vi "TriEdges-Box intersection test.vi"(1 "Triangle":T1, 2 "Box":T2={"Face 0"={"V0"=[], "V1"=[], "V2"=[], "V3"=[], "E0"=[], "E1"=[], "E2"=[], "E3"=[], "n^"=[], "nE0^"=[], "nE1^"=[], "nE2^"=[], "nE3^"=[]}, "Face 1"={"V0"=[], "V1"=[], "V2"=[], "V3"=[], "E0"=[], "E1"=[], "E2"=[], "E3"=[], "n^"=[], "nE0^"=[], "nE1^"=[], "nE2^"=[], "nE3^"=[]}, "Face 2"={"V0"=[], "V1"=[], "V2"=[], "V3"=[], "E0"=[], "E1"=[], "E2"=[], "E3"=[], "n^"=[], "nE0^"=[], "nE1^"=[], "nE2^"=[], "nE3^"=[]}, "Face 3"={"V0"=[], "V1"=[], "V2"=[], "V3"=[], "E0"=[], "E1"=[], "E2"=[], "E3"=[], "n^"=[], "nE0^"=[], "nE1^"=[], "nE2^"=[], "nE3^"=[]}, "Face 4"={"V0"=[], "V1"=[], "V2"=[], "V3"=[], "E0"=[], "E1"=[], "E2"=[], "E3"=[], "n^"=[], "nE0^"=[], "nE1^"=[], "nE2^"=[], "nE3^"=[]}, "Face 5"={"V0"=[], "V1"=[], "V2"=[], "V3"=[], "E0"=[], "E1"=[], "E2"=[], "E3"=[], "n^"=[], "nE0^"=[], "nE1^"=[], "nE2^"=[], "nE3^"=[]}, "Level"=-1, "Pmax"=[], "Pmin"=[], "Parent"=-1, "Child 1"=-1, "Child 2"=-1, "Child 3"=-1, "Child 4"=-1, "Child 5"=-1, "Child 6"=-1, "Child 7"=-1, "Child 8"=-1, "Triangles"=[], "is leaf node"=FALSE}) -> (0 "Intersection":bool)   [LabVIEW 2014]
uses:
  Typedefs/TreeNodeBox.ctl
  Typedefs/Quad.ctl
  Typedefs/Triangle.ctl
panel:
  # "PN 17/01/2015"
  # "Vertices"
  # "Edges"
  # "Unit normal"
  # "pre-store"
  # "Vertices"
  # "Edges"
  # "Unit normal"
  # "Edge unit normals"
  # "Vertices"
  # "Edges"
  # "Unit normal"
  # "Edge unit normals"
  # "Vertices"
  # "Edges"
  # "Unit normal"
  # "Edge unit normals"
  # "Vertices"
  # "Edges"
  # "Unit normal"
  # "Edge unit normals"
  # "Vertices"
  # "Edges"
  # "Unit normal"
  # "Edge unit normals"
  # "Vertices"
  # "Edges"
  # "Unit normal"
  # "Edge unit normals"
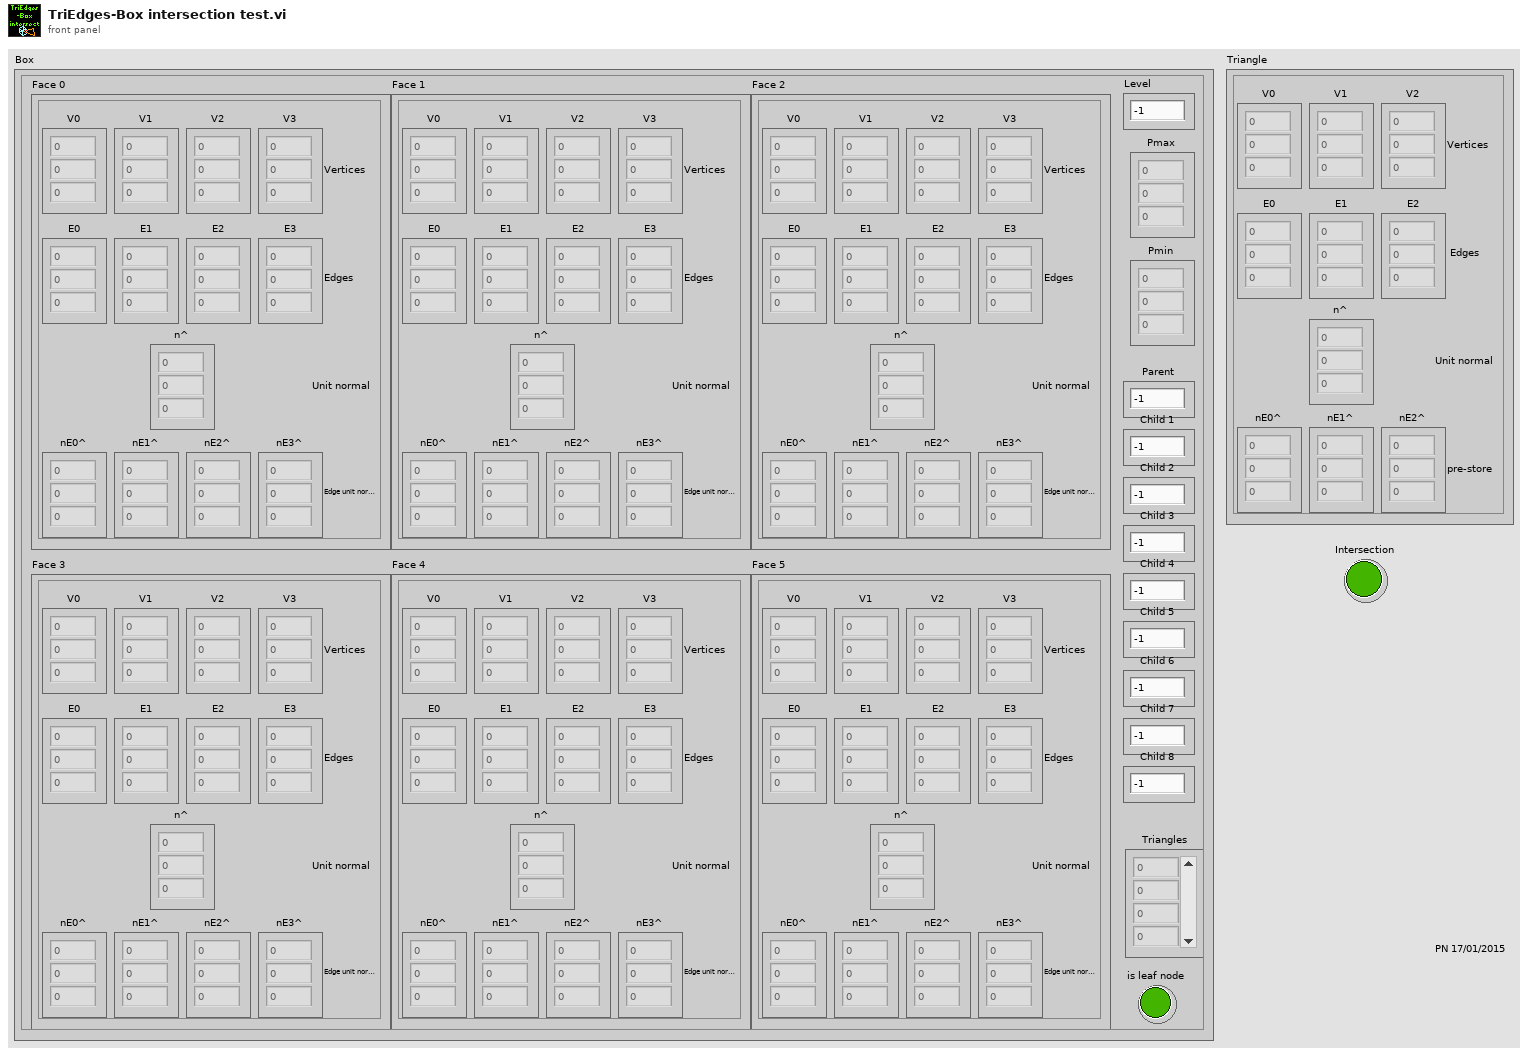
[diagram p1: front panel]
types:
  T1 = typedef "Triangle.ctl" = cluster{"V0":sgl[], "V1":sgl[], "V2":sgl[], "E0":sgl[], "E1":sgl[], "E2":sgl[], "n^":sgl[], "nE0^":sgl[], "nE1^":sgl[], "nE2^":sgl[]}
  T2 = typedef "TreeNodeBox.ctl" = cluster{"Face 0":T3, "Face 1":T3, "Face 2":T3, "Face 3":T3, "Face 4":T3, "Face 5":T3, "Level":i32, "Pmax":sgl[], "Pmin":sgl[], "Parent":i32, "Child 1":i32, "Child 2":i32, "Child 3":i32, "Child 4":i32, "Child 5":i32, "Child 6":i32, "Child 7":i32, "Child 8":i32, "Triangles":i32[], "is leaf node":bool}
  T3 = typedef "Quad.ctl" = cluster{"V0":sgl[], "V1":sgl[], "V2":sgl[], "V3":sgl[], "E0":sgl[], "E1":sgl[], "E2":sgl[], "E3":sgl[], "n^":sgl[], "nE0^":sgl[], "nE1^":sgl[], "nE2^":sgl[], "nE3^":sgl[]}
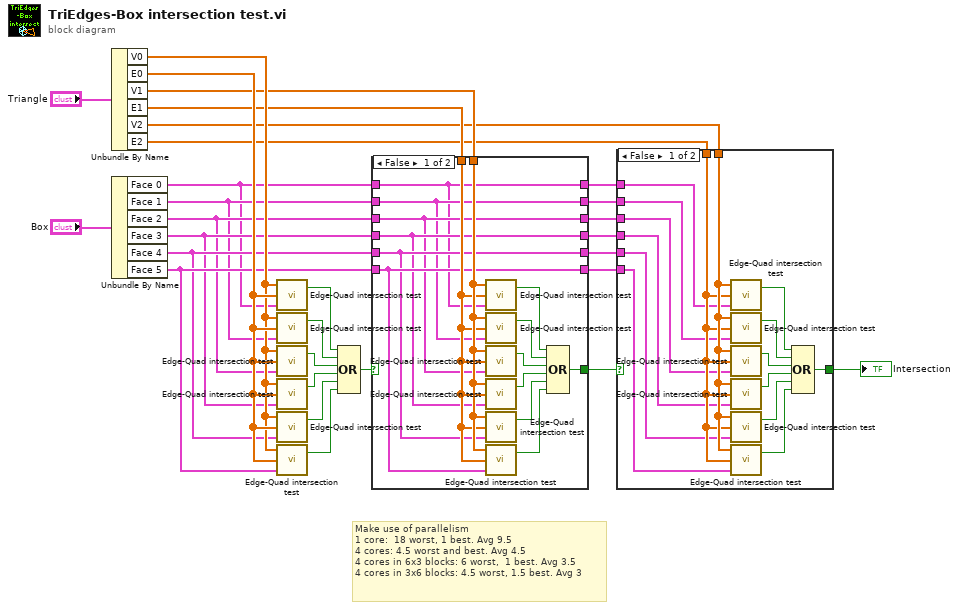
[diagram p0: block diagram]
diagram:
  # "Make use of parallelism\n1 core:  18 worst, 1 best. Avg 9.5\n4 cores: 4.5 worst and best. Avg 4.5\n4 cores in 6x3 blocks: 6 worst,  1 best. Avg 3.5\n4 cores in 3x6 blocks: 4.5 worst, 1.5 best. Avg 3"
  n1 = Unbundle By Name("Triangle") -> ("V0"=w26:sgl[], "E0"=w27:sgl[], "V1"=w18:sgl[], "E1"=w17:sgl[], "V2"=w15:sgl[], "E2"=w16:sgl[])
  n2 = Unbundle By Name("Box") -> ("Face 0"=w6:T3, "Face 1"=w7:T3, "Face 2"=w8:T3, "Face 3"=w9:T3, "Face 4"=w10:T3, "Face 5"=w12:T3)
  n3 = call "Edge-Quad intersection test.vi"("Quad"=w6, "Edge vector (not unit)"=w27, "Edge start point"=w26) -> ("Intersection"=w25:bool)  [unwired: 1 out]
  n4 = call "Edge-Quad intersection test.vi"("Quad"=w7, "Edge vector (not unit)"=w27, "Edge start point"=w26) -> ("Intersection"=w24:bool)  [unwired: 1 out]
  n5 = call "Edge-Quad intersection test.vi"("Quad"=w8, "Edge vector (not unit)"=w27, "Edge start point"=w26) -> ("Intersection"=w23:bool)  [unwired: 1 out]
  n6 = call "Edge-Quad intersection test.vi"("Quad"=w9, "Edge vector (not unit)"=w27, "Edge start point"=w26) -> ("Intersection"=w20:bool)  [unwired: 1 out]
  n7 = call "Edge-Quad intersection test.vi"("Quad"=w10, "Edge vector (not unit)"=w27, "Edge start point"=w26) -> ("Intersection"=w21:bool)  [unwired: 1 out]
  n8 = call "Edge-Quad intersection test.vi"("Quad"=w12, "Edge vector (not unit)"=w27, "Edge start point"=w26) -> ("Intersection"=w22:bool)  [unwired: 1 out]
  n9 = Compound Arithmetic op=OR(w25, w24, w23, w20, w21, w22) -> (w19:bool)
  n10 = case shown="False" w19 {
    selector: w19 -> [_ w51]
    tunnel: w18 -> [w38 _]
    tunnel: w17 -> [w37 _]
    tunnel: [w36 w51] -> w14
    tunnel: w12 -> [w35 w45]
    tunnel: [w35 w45] -> w11
    tunnel: w10 -> [w34 w46]
    tunnel: w9 -> [w33 w47]
    tunnel: w8 -> [w32 w48]
    tunnel: w7 -> [w31 w49]
    tunnel: w6 -> [w30 w50]
    tunnel: [w34 w46] -> w5
    tunnel: [w33 w47] -> w4
    tunnel: [w32 w48] -> w3
    tunnel: [w31 w49] -> w2
    tunnel: [w30 w50] -> w1
    frame False {
      n11 = call "Edge-Quad intersection test.vi"("Quad"=w30, "Edge vector (not unit)"=w37, "Edge start point"=w38) -> ("Intersection"=w39:bool)  [unwired: 1 out]
      n12 = call "Edge-Quad intersection test.vi"("Quad"=w31, "Edge vector (not unit)"=w37, "Edge start point"=w38) -> ("Intersection"=w40:bool)  [unwired: 1 out]
      n13 = call "Edge-Quad intersection test.vi"("Quad"=w32, "Edge vector (not unit)"=w37, "Edge start point"=w38) -> ("Intersection"=w41:bool)  [unwired: 1 out]
      n14 = call "Edge-Quad intersection test.vi"("Quad"=w33, "Edge vector (not unit)"=w37, "Edge start point"=w38) -> ("Intersection"=w44:bool)  [unwired: 1 out]
      n15 = call "Edge-Quad intersection test.vi"("Quad"=w34, "Edge vector (not unit)"=w37, "Edge start point"=w38) -> ("Intersection"=w43:bool)  [unwired: 1 out]
      n16 = call "Edge-Quad intersection test.vi"("Quad"=w35, "Edge vector (not unit)"=w37, "Edge start point"=w38) -> ("Intersection"=w42:bool)  [unwired: 1 out]
      n17 = Compound Arithmetic op=OR(w39, w40, w41, w44, w43, w42) -> (w36:bool)
    }
    frame True {
    }
  }
  n18 = case shown="False" w14 {
    selector: w14 -> [_ w67]
    tunnel: w15 -> [w60 _]
    tunnel: w16 -> [w59 _]
    tunnel: [w58 w67] -> w13
    tunnel: w11 -> [w57 _]
    tunnel: w5 -> [w56 _]
    tunnel: w4 -> [w55 _]
    tunnel: w3 -> [w54 _]
    tunnel: w2 -> [w53 _]
    tunnel: w1 -> [w52 _]
    frame False {
      n19 = call "Edge-Quad intersection test.vi"("Quad"=w52, "Edge vector (not unit)"=w59, "Edge start point"=w60) -> ("Intersection"=w61:bool)  [unwired: 1 out]
      n20 = call "Edge-Quad intersection test.vi"("Quad"=w53, "Edge vector (not unit)"=w59, "Edge start point"=w60) -> ("Intersection"=w62:bool)  [unwired: 1 out]
      n21 = call "Edge-Quad intersection test.vi"("Quad"=w54, "Edge vector (not unit)"=w59, "Edge start point"=w60) -> ("Intersection"=w63:bool)  [unwired: 1 out]
      n22 = call "Edge-Quad intersection test.vi"("Quad"=w55, "Edge vector (not unit)"=w59, "Edge start point"=w60) -> ("Intersection"=w66:bool)  [unwired: 1 out]
      n23 = call "Edge-Quad intersection test.vi"("Quad"=w56, "Edge vector (not unit)"=w59, "Edge start point"=w60) -> ("Intersection"=w65:bool)  [unwired: 1 out]
      n24 = call "Edge-Quad intersection test.vi"("Quad"=w57, "Edge vector (not unit)"=w59, "Edge start point"=w60) -> ("Intersection"=w64:bool)  [unwired: 1 out]
      n25 = Compound Arithmetic op=OR(w61, w62, w63, w66, w65, w64) -> (w58:bool)
    }
    frame True {
    }
  }
  "Intersection" <- w13
